vi "Gas Thermal Adv Tolerance Check.vi"(0 "Target RTDout-RTDin":dbl, 1 "Temperature +- Tolerance (F)":dbl=2.0, 5 "Inlet Temperature (F) - Target":dbl, 9 "Thermal Stabil Array":dbl[][](array[numeric]), 11 "error in (no error)":errorcluster) -> (4 "RTDOut-RTDin (Max-Min) - Bool":bool, 6 "RTDout (Max-Min) Bool":bool, 8 "RTDout >= Target":bool, 10 "RTDin (Max-Min) Bool":bool, 15 "error out":errorcluster)   [LabVIEW 2023]
uses:
  <vilib>/numeric/Random Number (Range) DBL.vi
panel:
  out "Target RTDout":dbl
  in  "Debug":bool
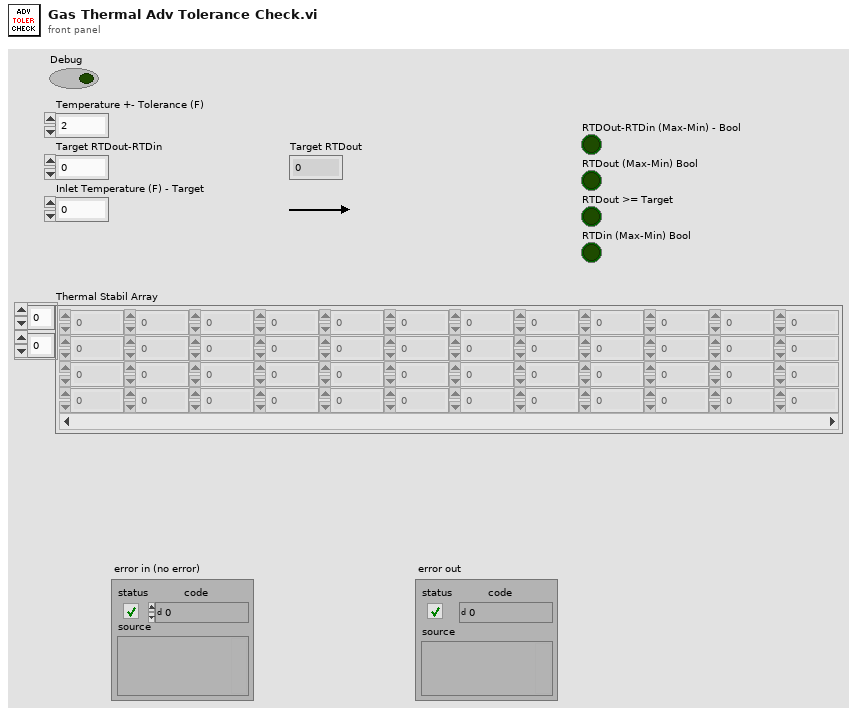
[diagram p1: front panel]
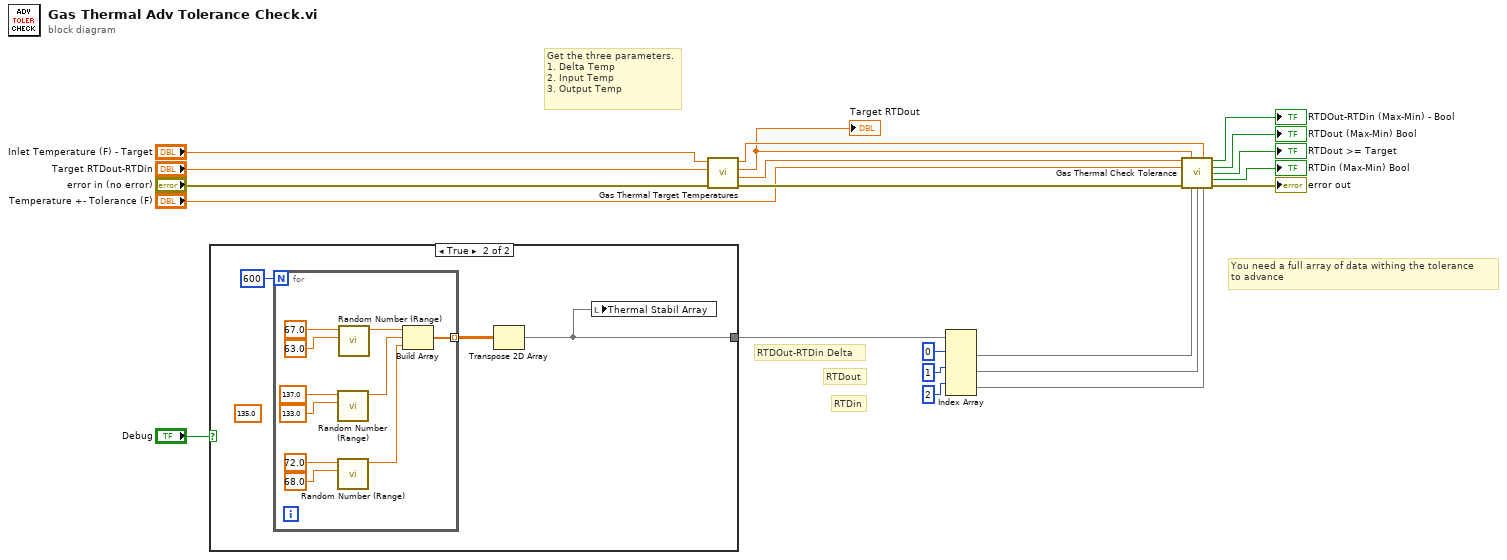
[diagram p0: block diagram]
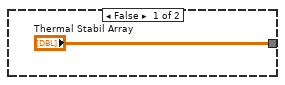
[diagram p2: hidden frame]
diagram:
  # "Get the three parameters.\n1. Delta Temp\n2. Input Temp\n3. Output Temp"
  # "You need a full array of data withing the tolerance \nto advance"
  # "RTDout"
  # "RTDOut-RTDin Delta"
  # "RTDin"
  n1 = case shown="True" "Debug" {
    tunnel: ["Thermal Stabil Array" w23] -> w17
    frame False {
    }
    frame True {
      (unwired) 135.0 ("lower bound (0)")
      n2 = for {
        N: 600 -> [_]
        tunnel: [w26] -> w24 mode=indexing
        n3 = call-poly <vilib>:"Random Number (Range).vi"("lower bound (0)"=133.0, "upper bound (100)"=137.0) -> ("number"=w28:dbl)  [unwired: 9 in]
        n4 = call-poly <vilib>:"Random Number (Range).vi"("lower bound (0)"=68.0, "upper bound (100)"=72.0) -> ("number"=w27:dbl)  [unwired: 9 in]
        n5 = call-poly <vilib>:"Random Number (Range).vi"("lower bound (0)"=63.0, "upper bound (100)"=67.0) -> ("number"=w29:dbl)  [unwired: 9 in]
        n6 = Build Array(w29, w28, w27) -> (w26:dbl[])
      }
      n7 = Transpose 2D Array(2D array=w24) -> (transposed array=w23:dbl[][])
      n8 = local write "Thermal Stabil Array"(w23) -> ()
    }
  }
  n9 = call "Gas Thermal Target Temperatures.vi"("error in (no error)"="error in (no error)", "Target RTDout-RTDin in"="Target RTDout-RTDin", "Inlet Temperature (F) - Target in"="Inlet Temperature (F) - Target") -> ("error out"=w7:errorcluster, "Target RTDout-RTDin out"=w14:dbl, "Target RTDout"=w11:dbl, "Target Inlet Temperature (F)"=w13:dbl)  [unwired: 5 in]
  "Target RTDout" <- w11
  n10 = Index Array(array=w17, index (row) #1=0 ("index (row)"), index (row) #2=1 ("index (row)"), index (row) #3=2 ("index (row)")) -> (element #1=w3:dbl[], element #2=w4:dbl[], element #3=w12:dbl[])  [unwired: 3 in]
  n11 = call "Gas Thermal Check Tolerance.vi"("Target RTDout-RTDin in"=w14, "Target RTDout"=w11, "Target Inlet Temperature (F)"=w13, "Temperature +- Tolerance (F)"="Temperature +- Tolerance (F)", "error in (no error)"=w7, "RTDOut-RTDin Delta"=w3, "RTDout"=w4, "RTDin"=w12) -> ("RTDOut-RTDin (Max-Min) - Bool"=→"RTDOut-RTDin (Max-Min) - Bool":bool, "RTDout (Max-Min) Bool"=→"RTDout (Max-Min) Bool":bool, "RTDout >= Target"=→"RTDout >= Target":bool, "RTDin (Max-Min) Bool"=→"RTDin (Max-Min) Bool":bool, "error out"=→"error out":errorcluster)  [unwired: 3 in]
